vi "VariantTest.vi"() -> ()   [LabVIEW 2016, in "M1M3SupportEUI_Views.lvlib"]
uses:
  M1M3SupportEUI_Views.lvlib
panel:
  out "T6":dbl
  out "T5":dbl
  out "T4":dbl
  out "T3":dbl
  out "T2":dbl
  out "T1":dbl
  # "3"
  # "1"
  # "2"
  # "6"
  # "4"
  # "5"
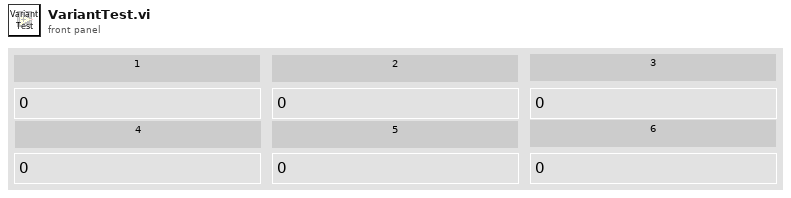
[diagram p1: front panel]
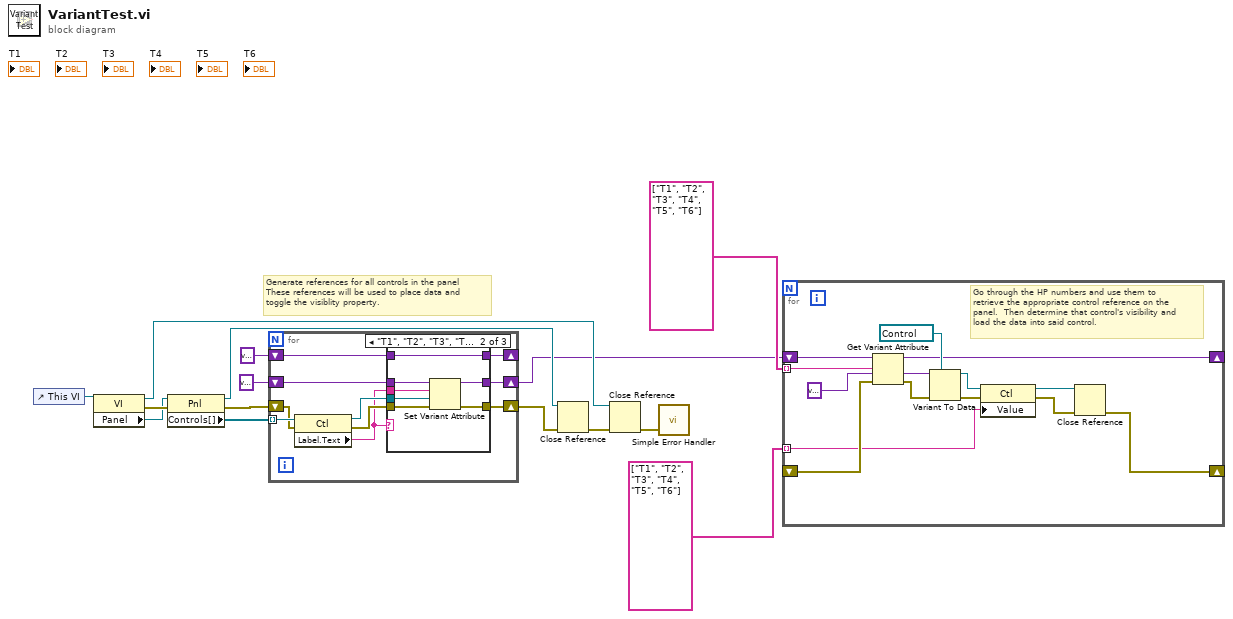
[diagram p0: block diagram]
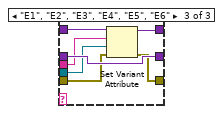
[diagram p3: hidden frame]
diagram:
  # "Generate references for all controls in the panel\nThese references will be used to place data and\ntoggle the visiblity property."
  n1 = control-ref of="This VI"() -> (w14:refnum<vi>)
  n2 = property class="VI"(reference=w14) -> (reference out=w4:refnum<vi>, error out=w13:errorcluster, "Panel"=w12:refnum<vi>)  [unwired: 1 in]
  n3 = property class="Pnl"(reference=w12, error in=w13) -> (reference out=w6:refnum<vi>, error out=w9:errorcluster, "Controls[]"=w11:refnum<vi>[])
  n4 = for {
    tunnel: w11 -> [w25] mode=indexing
    shift-right: [w22] -> w1
    shift-left: variant -> [w24]
    shift-right: [w19] -> w7
    shift-left: w9 -> [w21]
    shift-right: [w17] -> _
    shift-left: variant -> [w18]
    n5 = property class="Ctl"(reference=w25, error in=w21) -> (reference out=w23:refnum<vi>, error out=w20:errorcluster, "Label.Text"=w16:string)
    n6 = case shown="\"T1\", \"T2\", \"T3\", \"T4\", \"T5\", \"T6\"" w16 {
      tunnel: w24 -> [w27 w35 w40]
      tunnel: w16 -> [_ w34 w39]
      tunnel: w23 -> [_ w33 w38]
      tunnel: [w27 w32 w40] -> w22
      tunnel: w20 -> [w26 w31 w37]
      tunnel: [w26 w30 w36] -> w19
      tunnel: w18 -> [w28 w29 w42]
      tunnel: [w28 w29 w41] -> w17
      frame "", Default {
      }
      frame "T1", "T2", "T3", "T4", "T5", "T6" {
        n7 = Set Variant Attribute(Variant=w35, name=w34, value=w33, error in=w31) -> (Variant out=w32:variant, error out=w30:errorcluster)  [unwired: 1 out]
      }
      frame "E1", "E2", "E3", "E4", "E5", "E6" {
        n8 = Set Variant Attribute(Variant=w42, name=w39, value=w38, error in=w37) -> (Variant out=w41:variant, error out=w36:errorcluster)  [unwired: 1 out]
      }
    }
  }
  n9 = Close Reference(reference=w6, error in (no error)=w7) -> (error out=w8:errorcluster)
  n10 = Close Reference(reference=w4, error in (no error)=w8) -> (error out=w5:errorcluster)
  n11 = call <vilib>:"Simple Error Handler.vi"("error in (no error)"=w5) -> ()  [unwired: 4 in, 5 out]
  n12 = for {
    shift-right: [w48] -> _
    shift-left: _ -> [w50]
    tunnel: string[] ["T1", "T2", "T3", "T4", "T5", "T6"] -> [w45] mode=indexing
    tunnel: string[] ["T1", "T2", "T3", "T4", "T5", "T6"] -> [w44] mode=indexing
    shift-right: [w43] -> _
    shift-left: w1 -> [w46]
    # "Go through the HP numbers and use them to \nretrieve the appropriate control reference on the\npanel.  Then determine that control's visibility and\nload the data into said control."
    n13 = Get Variant Attribute(Variant=w46, name=w45, default value (empty Variant)=variant ("default value (empty variant)"), error in=w50) -> (duplicate Variant=w43:variant, value=w54:variant, error out=w53:errorcluster)  [unwired: 1 out]
    n14 = Variant To Data(error in=w53, type=refnum<vi> refnum ("reference out"), Variant=w54) -> (data=w52:refnum<vi>, error out=w51:errorcluster)
    n15 = property class="Ctl"(reference=w52, error in=w51, "Value"=w44) -> (reference out=w47:refnum<vi>, error out=w49:errorcluster)
    n16 = Close Reference(reference=w47, error in (no error)=w49) -> (error out=w48:errorcluster)
  }
